vi "Plot Editor_Store to Controls.vi"(8 "Error In":errorcluster, 10 "Control Refnums":refnum<vi>[](array[refnum]), 11 "Plot Editor Internal Data in":T1) -> (0 "Error Out":errorcluster, 3 "Plot Editor Internal Data out":T1)   [LabVIEW 2019, in "Plot Editor.lvlib"]
uses:
  Plot Editor.lvlib
  Plot Editor Internal Variables.ctl
  XY Graph Plot Properties.ctl
panel:
  in  "Array":refnum<vi>
  in  "Numeric":refnum<vi>
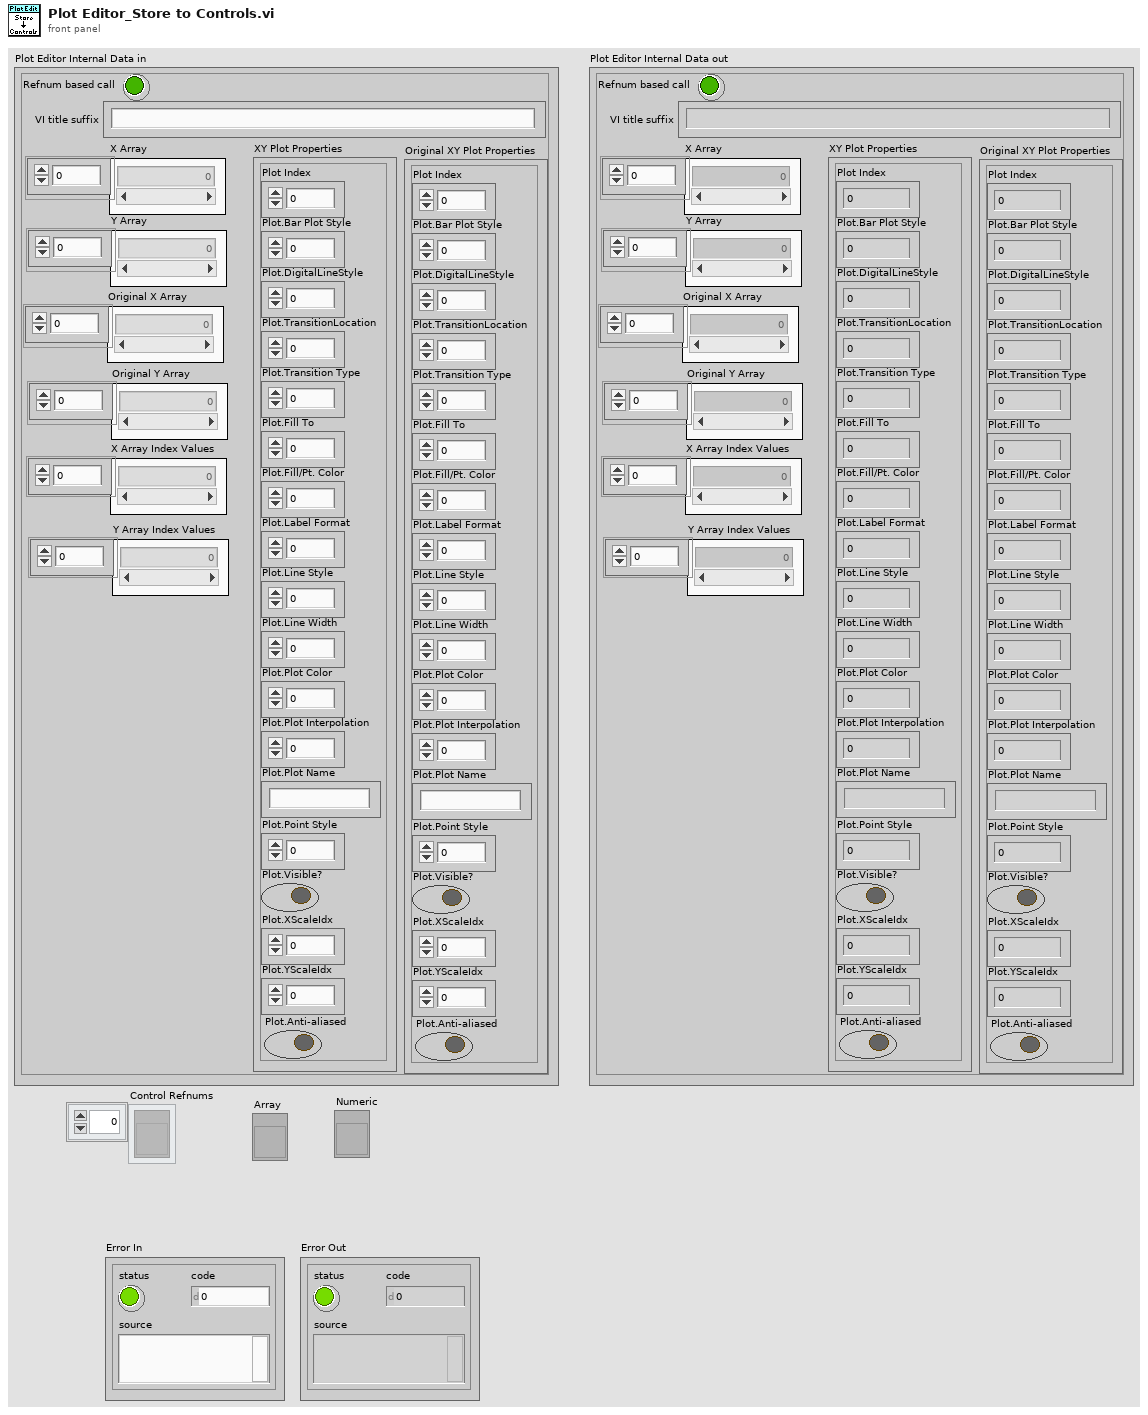
[diagram p1: front panel]
types:
  T1 = typedef "Plot Editor.lvlib/Plot Editor Internal Variables.ctl" = cluster{"X Array":dbl[], "Y Array":dbl[], "XY Plot Properties":T2, "X Array Index Values":u32[], "Y Array Index Values":u32[], "Original XY Plot Properties":T2, "Original X Array":dbl[], "Original Y Array":dbl[], "VI title suffix":string, "Refnum based call":bool}
  T2 = typedef "XY Graph Plot Properties.ctl" = cluster{"Plot Index":i32, "Plot.Bar Plot Style":u8, "Plot.DigitalLineStyle":u8, "Plot.TransitionLocation":u8, "Plot.Transition Type":u8, "Plot.Fill To":i16, "Plot.Fill/Pt. Color":u32, "Plot.Label Format":u8, "Plot.Line Style":u8, "Plot.Line Width":u8, "Plot.Plot Color":u32, "Plot.Plot Interpolation":u8, "Plot.Plot Name":string, "Plot.Point Style":u8, "Plot.Visible?":bool, "Plot.XScaleIdx":u32, "Plot.YScaleIdx":u32, "Plot.Anti-aliased":bool}
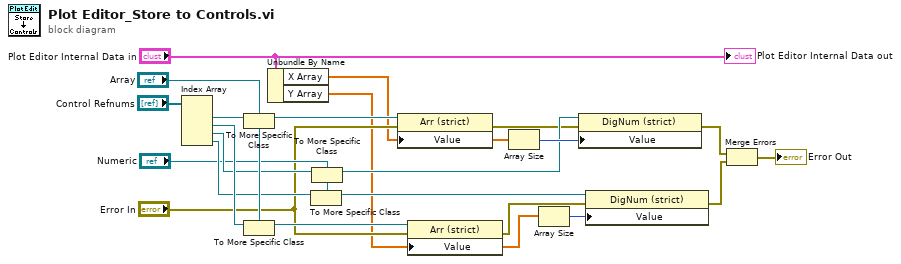
[diagram p0: block diagram]
diagram:
  n1 = Index Array(array="Control Refnums") -> (element #1=w19:refnum<vi>, element #2=w17:refnum<vi>, element #3=w14:refnum<vi>, element #4=w12:refnum<vi>)  [unwired: 4 in]
  n2 = To More Specific Class(target class="Array", reference=w19) -> (specific class reference=w18:refnum<vi>)  [unwired: 1 in, 1 out]
  n3 = To More Specific Class(target class="Array", reference=w17) -> (specific class reference=w15:refnum<vi>)  [unwired: 1 in, 1 out]
  n4 = Unbundle By Name("Plot Editor Internal Data in") -> ("X Array"=w2:dbl[], "Y Array"=w1:dbl[])
  n5 = To More Specific Class(target class="Numeric", reference=w12) -> (specific class reference=w10:refnum<vi>)  [unwired: 1 in, 1 out]
  n6 = To More Specific Class(target class="Numeric", reference=w14) -> (specific class reference=w13:refnum<vi>)  [unwired: 1 in, 1 out]
  n7 = property class="Arr (strict)"(reference=w18, error in="Error In", "Value"=w2) -> (error out=w8:errorcluster)  [unwired: 1 out]
  n8 = property class="Arr (strict)"(reference=w15, error in="Error In", "Value"=w1) -> (error out=w7:errorcluster)  [unwired: 1 out]
  n9 = Array Size(array=w2) -> (size(s)=w21:i32)
  n10 = Array Size(array=w1) -> (size(s)=w22:i32)
  n11 = property class="DigNum (strict)"(reference=w13, error in=w8, "Value"=w21) -> (error out=w6:errorcluster)  [unwired: 1 out]
  n12 = property class="DigNum (strict)"(reference=w10, error in=w7, "Value"=w22) -> (error out=w4:errorcluster)  [unwired: 1 out]
  n13 = Merge Errors(w6, w4) -> (→"Error Out":errorcluster)
  "Plot Editor Internal Data out" <- "Plot Editor Internal Data in"
